vi "Pagina diagnostica.vi"(3 "error in (no error)":errorcluster) -> (9 "pagina out":i16=255, 10 "error out (no error)":errorcluster)   [LabVIEW 2022 SP3]
uses:
  <vilib>/Platform/TimedLoop/XDataNode/timing_clust.ctl
  <vilib>/Platform/TimedLoop/XDataNode/nitl_modes.ctl
  <vilib>/Platform/TimedLoop/XDataNode/wakeup.ctl
  Labview/Globali.vi
  <vilib>/platform/TimedLoop/XDataNode/XDataNode.xnode
  <vilib>/Platform/TimedLoop/XDataNode/XDNodeRunTimeDep.lvlib
panel:
  in  "226. 0":sgl min=0 format="%.2f"
  in  "230. 0":sgl min=0 format="%.2f"
  in  "Verniciato":bool
  out "CICLO_IN_CORSO":bool
  out "S_SCARTO":bool
  out "S_PAUSA":bool
  out "Cicli_macchina":u16
  in  "2. 8":bool
  in  "2. 7":bool
  out "S_CANCELLI_APERTI":bool
  out "S_CANCELLI_CHIUSI":bool
  out "S_CANCELLO_CHIUSURA":bool
  out "S_CANCELLO_APERTURA":bool
  out "V_SOVRAPRESSIONE_DX":sgl format="%.2f"
  out "V_SOVRAPRESSIONE_SX":sgl format="%.2f"
  out "CALIBRAZIONE_TORSIOMETRO":bool
  in  "2. 6":bool
  out "S_CARRO_IN_POSIZ_RP3000":bool
  out "S_FILTRO_INTASATO_PROT35":bool
  out "S_FILTRO_INTASATO_RICIRC":bool
  in  "2. 5":bool
  out "S_CANCELLO_DX_APERTO":bool
  out "S_CANCELLO_SX_CHIUSO":bool
  out "S_CANCELLO_DX_CHIUSO":bool
  out "S_AUX_ON":bool
  out "S_PRESSOSTATO_ARIA":bool
  out "S_CANCELLO_SX_APERTO":bool
  out "S_CANCELLO_SX_SBLOCCATO":bool
  out "S_CANCELLO_DX_SBLOCCATO":bool
  out "S_TRAZIONE_INSERITA":bool
  out "S_SCARICO_A_LAV":bool
  out "S_SCARICO_A_RIP":bool
  out "S_CARRELLO_10W30":bool
  out "S_CARRELLO_W90":bool
  out "S_CARRELLO_PROT35":bool
  out "S_SCARICO_B_LAV":bool
  out "S_SCARICO_B_RIP":bool
  out "S_CARRO_IN_POSIZ_AAT":bool
  out "S_MOTORE_FERMO":bool
  out "C_APERTURA_CANCELLI":bool
  out "C_START_PROVA":bool
  out "C_RESET":bool
  out "C_CHIUSURA_CANCELLI":bool
  out "C_FASE_SUCCESSIVA":bool
  out "S_ALLARME_INVERTER":bool
  out "S_LIVELLO_MIN_10W30":bool
  out "S_LIVELLO_MIN_W90":bool
  out "S_LIVELLO_MIN_PROT35":bool
  out "S_FILTRO_INTASATO_10W30":bool
  out "S_FILTRO_INTASATO_W90":bool
  out "S_PERDITA_10W30":bool
  out "S_PERDITA_W90":bool
  out "S_PERDITA_PROT35":bool
  out "S_TERMICA_10W30":bool
  out "S_TERMICA_W90":bool
  out "S_TERMICA_PROT35":bool
  out "S_TERMICA_RICIRCOLO":bool
  out "CARICO_ARIA_6_BAR":bool
  out "SCARICO_ARIA_6_BAR":bool
  out "CARICO_PRESSURIZZ":bool
  out "S_PERDITA_VASCA_RACCOLT":bool
  out "SCARICO_PRESSURIZZ":bool
  out "RICIRCOLO_OLIO":bool
  out "ACCENSIONE_AZIONAMENTO":bool
  out "START_MOTORE":bool
  out "POMPA_RICIRCOLO":bool
  out "SCARICO_B":bool
  out "EROGAZIONE_10W30":bool
  out "EROGAZIONE_W90":bool
  out "CHIUSURA_CANCELLI":bool
  out "APERTURA_CANCELLI":bool
  out "SCARICO_A":bool
  out "EROGAZIONE_PROT35":bool
  out "ROTAZIONE_SX":bool
  out "SBLOCCO_CANCELLI":bool
  out "LAMPADA_TRAZIONE_ON":bool
  out "POMPA_10W30":bool
  out "POMPA_W90":bool
  out "POMPA_PROT35":bool
  out "LAMPADA_ROSSA":bool
  out "LAMPADA_GIALLA":bool
  out "LAMPADA_VERDE":bool
  out "CICALINO":bool
  out "S_MAN":bool
  out "S_AUTO":bool
  out "mA_RICIRCOLO_OK":bool
  out "mA_RISCALDAMENTO_OK":bool
  out "mA_PRESS_INSERZ_ASSE_OK":bool
  out "mA_TRAZIONE_INSERITA":bool
  out "mA_TRAZIONE_DISINSERITA":bool
  out "mA_RODAGGIO_OK":bool
  out "mA_COPPIA_1_FUN_OK":bool
  out "mA_RICIRCOLO_1_FUN_OK":bool
  out "mA_COPPIA_2_FUN_OK":bool
  out "mA_RICIRCOLO_2_FUN_OK":bool
  out "mA_COPPIA_3_FUN_OK":bool
  out "S_ALLARME":bool
  out "mA_RICIRCOLO_3_FUN_OK":bool
  out "mA_GONFIAGGIO_OK":bool
  out "mA_PERDITE_DX_OK":bool
  out "mA_PERDITE_SX_OK":bool
  out "mA_COPPIA_4_FUN_OK":bool
  out "mA_RICIRCOLO_4_FUN_OK":bool
  out "mA_COPPIA_5_FUN_OK":bool
  out "mA_RICIRCOLO_5_FUN_OK":bool
  out "mA_PRESS_PRESSURIZZ_OK":bool
  out "mA_PRESSURIZZ_DX_OK":bool
  out "mA_PRESSURIZZ_SX_OK":bool
  out "Messaggi":u16
  out "Segnalazioni":u16
  out "Allarmi":u16
  out "Fase_collaudo":u16
  out "V_PORT_RICIRC_4_FUN_AAT2":sgl format="%.2f"
  out "V_PRES_OLIO_RICIRC_4_FUN":sgl format="%.2f"
  out "V_TEMP_CUSCIN_4_FUN_AAT":sgl format="%.2f"
  out "V_COPPIA_4_FUN":sgl format="%.2f"
  out "V_TEMP_OLIO_4_FUN":sgl format="%.2f"
  out "V_PORT_RICIRC_2_FUN_AAT2":sgl format="%.2f"
  out "V_PRES_OLIO_RICIRC_2_FUN":sgl format="%.2f"
  out "V_TEMP_CUSCIN_2_FUN_AAT":sgl format="%.2f"
  out "V_COPPIA_2_FUN":sgl format="%.2f"
  out "V_TEMP_OLIO_2_FUN":sgl format="%.2f"
  out "V_PERDITA_PRESSURIZZ_SX":sgl format="%.2f"
  out "V_PERDITA_PRESSURIZZ_DX":sgl format="%.2f"
  out "V_PERDITA_GONFIAGGIO_SX":sgl format="%.2f"
  out "V_PERDITA_GONFIAGGIO_DX":sgl format="%.2f"
  out "V_PRESS_PRESSURIZZ":sgl format="%.2f"
  out "V_PORT_RICIRC_5_FUN_AAT2":sgl format="%.2f"
  out "V_PRES_OLIO_RICIRC_5_FUN":sgl format="%.2f"
  out "V_TEMP_CUSCIN_5_FUN_AAT":sgl format="%.2f"
  out "V_COPPIA_5_FUN":sgl format="%.2f"
  out "V_TEMP_OLIO_5_FUN":sgl format="%.2f"
  out "V_PORT_RICIRC_3_FUN_AAT2":sgl format="%.2f"
  out "V_PRES_OLIO_RICIRC_3_FUN":sgl format="%.2f"
  out "V_TEMP_CUSCIN_3_FUN_AAT":sgl format="%.2f"
  out "V_COPPIA_3_FUN":sgl format="%.2f"
  out "V_TEMP_OLIO_3_FUN":sgl format="%.2f"
  out "V_PORT_RICIRC_1_FUN_AAT2":sgl format="%.2f"
  out "V_PRES_OLIO_RICIRC_1_FUN":sgl format="%.2f"
  out "V_TEMP_CUSCIN_1_FUN_AAT":sgl format="%.2f"
  out "V_COPPIA_1_FUN":sgl format="%.2f"
  out "V_TEMP_OLIO_1_FUN":sgl format="%.2f"
  out "V_TEMP_OLIO_10W90":sgl format="%.2f"
  out "V_TEMP_OLIO_10W30":sgl format="%.2f"
  out "V_TEMP_OLIO_RP3000":sgl format="%.2f"
  out "V_TEMP_OLIO_AAT_1_3_4":sgl format="%.2f"
  out "V_TEMP_OLIO_AAT_2":sgl format="%.2f"
  out "V_TEMP_OLIO_ROD":sgl format="%.2f"
  out "V_GONFIAGGIO_STAB":sgl format="%.2f"
  out "VI_COPPIA_MOT":u16
  out "VO_VEL_MOT":u16
  out "VI_VEL_MOT":u16
  out "V_COPPIA_ASSE_TRASCINAM":sgl format="%.2f"
  out "V_PORTATA_RICIRCOLO":sgl format="%.2f"
  out "V_PRESS_OLIO_RICIRCOLO":sgl format="%.2f"
  out "V_PRESSURIZZAZIONE":sgl format="%.2f"
  out "V_PRESS_ARIA_6_BAR":sgl format="%.2f"
  out "V_TEMP_CUSCINETTO_AAT":sgl format="%.2f"
  out "V_TEMP_AMBIENTE":sgl format="%.2f"
  in  "0. 0":bool
  in  "0. 1":bool
  in  "0. 2":bool
  in  "0. 3":bool
  in  "0. 4":bool
  in  "0. 5":bool
  in  "0. 6":bool
  in  "0. 7":bool
  in  "1. 0":bool
  in  "1. 1":bool
  in  "1. 2":bool
  in  "1. 3":bool
  in  "1. 4":bool
  in  "1. 5":bool
  in  "1. 6":bool
  in  "1. 7":bool
  in  "2. 0":bool
  in  "2. 1":bool
  in  "2. 2":bool
  in  "2. 3":bool
  in  "2. 4":bool
  in  "4. 0":i16(ring) items=["PRODOTTO", "RP3000", "AAT 2", "AAT 1 3 4"]
  in  "6. 0":i16(ring) items=["TIPO", "PRODUZIONE", "RICAMBIO"]
  in  "8. 0":i16 min=0 max=3000
  in  "12. 0":sgl min=0 format="%.2f"
  in  "16. 0":i16 min=0
  in  "22. 0":sgl min=0 format="%.2f"
  in  "26. 0":sgl min=0 format="%.2f"
  in  "32. 0":sgl min=0 format="%.2f"
  in  "36. 0":sgl min=0 format="%.2f"
  in  "44. 0":i16 min=0
  in  "50. 0":i16 min=0
  in  "56. 0":i16 min=0
  in  "62. 0":i16 min=0
  in  "68. 0":i16 min=0
  in  "72. 0":sgl min=0 format="%.2f"
  in  "76. 0":sgl min=0 format="%.2f"
  in  "80. 0":sgl min=0 format="%.2f"
  in  "84. 0":i16 min=0
  in  "88. 0":sgl min=0 format="%.2f"
  in  "92. 0":sgl min=0 format="%.2f"
  in  "96. 0":sgl min=0 format="%.2f"
  in  "100. 0":i16 min=0
  in  "104. 0":sgl min=0 format="%.2f"
  in  "108. 0":sgl min=0 format="%.2f"
  in  "112. 0":sgl min=0 format="%.2f"
  in  "116. 0":i16 min=0
  in  "120. 0":sgl min=0 format="%.2f"
  in  "124. 0":sgl min=0 format="%.2f"
  in  "128. 0":sgl min=0 format="%.2f"
  in  "134. 0":sgl min=0 format="%.2f"
  in  "138. 0":sgl min=0 format="%.2f"
  in  "144. 0":i16 min=0
  in  "148. 0":i16 min=0
  in  "154. 0":i16 min=0
  in  "160. 0":sgl min=0 format="%.2f"
  in  "164. 0":sgl min=0 format="%.2f"
  in  "168. 0":sgl min=0 format="%.2f"
  in  "172. 0":i16 min=0
  in  "176. 0":sgl min=0 format="%.2f"
  in  "180. 0":sgl min=0 format="%.2f"
  in  "184. 0":sgl min=0 format="%.2f"
  in  "190. 0":sgl min=0 format="%.2f"
  in  "194. 0":sgl min=0 format="%.2f"
  in  "200. 0":i16 min=0
  in  "206. 0":i16 min=0
  in  "212. 0":i16 min=0
  in  "20. 0":u16
  in  "30. 0":u16
  in  "40. 0":u16
  in  "42. 0":u16
  in  "48. 0":u16
  in  "54. 0":u16
  in  "60. 0":u16
  in  "66. 0":u16
  in  "132. 0":u16
  in  "142. 0":u16
  in  "152. 0":u16
  in  "158. 0":u16
  in  "188. 0":u16
  in  "198. 0":u16
  in  "204. 0":u16
  in  "210. 0":u16
  in  "216. 0":u16
  in  "218. 0":u16
  out "PLC->PC":string[][](table)=[["WORD 0", "", "WORD 32", "", "WORD 64", "", "WORD 96", ""], ["WORD 1", "", "WORD 33", "", "WORD 65", "", "WORD 97", ""], ["WORD 2", "", "WORD 34", "", "WORD 66", "", "WORD 98", ""], ["WORD 3", "", "WORD 35", "", "WORD 67", "", "WORD 99", ""], ["WORD 4", "", "WORD 36", "", "WORD 68", "", "WORD 100", ""], ["WORD 5", "", "WORD 37", "", "WORD 69", "", "WORD 101", ""], ["WORD 6", "", "WORD 38", "", "WORD 70", "", "WORD 102", ""], ["WORD 7", "", "WORD 39", "", "WORD 71", "", "WORD 103", ""], ["WORD 8", "", "WORD 40", "", "WORD 72", "", "WORD 104", ""], ["WORD 9", "", "WORD 41", "", "WORD 73", "", "WORD 105", ""], ["WORD 10", "", "WORD 42", "", "WORD 74", "", "WORD 106", ""], ["WORD 11", "", "WORD 43", "", "WORD 75", "", "WORD 107", ""], ["WORD 12", "", "WORD 44", "", "WORD 76", "", "WORD 108", ""], ["WORD 13", "", "WORD 45", "", "WORD 77", "", "WORD 109", ""], ["WORD 14", "", "WORD 46", "", "WORD 78", "", "WORD 110", ""], ["WORD 15", "", "WORD 47", "", "WORD 79", "", "WORD 111", ""], ["WORD 16", "", "WORD 48", "", "WORD 80", "", "WORD 112", ""], ["WORD 17", "", "WORD 49", "", "WORD 81", "", "WORD 113", ""], ["WORD 18", "", "WORD 50", "", "WORD 82", "", "WORD 114", ""], ["WORD 19", "", "WORD 51", "", "WORD 83", "", "WORD 115", ""], ["WORD 20", "", "WORD 52", "", "WORD 84", "", "WORD 116", ""], ["WORD 21", "", "WORD 53", "", "WORD 85", "", "WORD 117", ""], ["WORD 22", "", "WORD 54", "", "WORD 86", "", "WORD 118", ""], ["WORD 23", "", "WORD 55", "", "WORD 87", "", "WORD 119", ""], ["WORD 24", "", "WORD 56", "", "WORD 88", "", "WORD 120", ""], ["WORD 25", "", "WORD 57", "", "WORD 89", "", "WORD 121", ""], ["WORD 26", "", "WORD 58", "", "WORD 90", "", "WORD 122", ""], ["WORD 27", "", "WORD 59", "", "WORD 91", "", "WORD 123", ""], ["WORD 28", "", "WORD 60", "", "WORD 92", "", "WORD 124", ""], ["WORD 29", "", "WORD 61", "", "WORD 93", "", "WORD 125", ""], ["WORD 30", "", "WORD 62", "", "WORD 94", "", "WORD 126", ""], ["WORD 31", "", "WORD 63", "", "WORD 95", "", "WORD 127", ""], ["", "", "", "", "", "", "", ""], ["", "", "", "", "", "", "", ""], ["", "", "", "", "", "", "", ""], ["", "", "", "", "", "", "", ""], ["", "", "", "", "", "", "", ""], ["", "", "", "", "", "", "", ""], ["", "", "", "", "", "", "", ""], ["", "", "", "", "", "", "", ""], ["", "", "", "", "", "", "", ""], ["", "", "", "", "", "", "", ""], ["", "", "", "", "", "", "", ""], ["", "", "", "", "", "", "", ""], ["", "", "", "", "", "", "", ""], ["", "", "", "", "", "", "", ""], ["", "", "", "", "", "", "", ""], ["", "", "", "", "", "", "", ""], ["", "", "", "", "", "", "", ""], ["", "", "", "", "", "", "", ""], ["", "", "", "", "", "", "", ""], ["", "", "", "", "", "", "", ""], ["", "", "", "", "", "", "", ""], ["", "", "", "", "", "", "", ""], ["", "", "", "", "", "", "", ""], ["", "", "", "", "", "", "", ""], ["", "", "", "", "", "", "", ""], ["", "", "", "", "", "", "", ""], ["", "", "", "", "", "", "", ""], ["", "", "", "", "", "", "", ""], ["", "", "", "", "", "", "", ""], ["", "", "", "", "", "", "", ""], ["", "", "", "", "", "", "", ""], ["", "", "", "", "", "", "", ""], ["", "", "", "", "", "", "", ""], ["", "", "", "", "", "", "", ""], ["", "", "", "", "", "", "", ""], ["", "", "", "", "", "", "", ""], ["", "", "", "", "", "", "", ""], ["", "", "", "", "", "", "", ""], ["", "", "", "", "", "", "", ""], ["", "", "", "", "", "", "", ""], ["", "", "", "", "", "", "", ""], ["", "", "", "", "", "", "", ""], ["", "", "", "", "", "", "", ""], ["", "", "", "", "", "", "", ""], ["", "", "", "", "", "", "", ""], ["", "", "", "", "", "", "", ""], ["", "", "", "", "", "", "", ""], ["", "", "", "", "", "", "", ""], ["", "", "", "", "", "", "", ""], ["", "", "", "", "", "", "", ""], ["", "", "", "", "", "", "", ""], ["", "", "", "", "", "", "", ""], ["", "", "", "", "", "", "", ""], ["", "", "", "", "", "", "", ""], ["", "", "", "", "", "", "", ""], ["", "", "", "", "", "", "", ""], ["", "", "", "", "", "", "", ""], ["", "", "", "", "", "", "", ""], ["", "", "", "", "", "", "", ""], ["", "", "", "", "", "", "", ""], ["", "", "", "", "", "", "", ""], ["", "", "", "", "", "", "", ""], ["", "", "", "", "", "", "", ""], ["", "", "", "", "", "", "", ""], ["", "", "", "", "", "", "", ""], ["", "", "", "", "", "", "", ""], ["", "", "", "", "", "", "", ""], ["", "", "", "", "", "", "", ""], ["", "", "", "", "", "", "", ""], ["", "", "", "", "", "", "", ""], ["", "", "", "", "", "", "", ""], ["", "", "", "", "", "", "", ""], ["", "", "", "", "", "", "", ""], ["", "", "", "", "", "", "", ""], ["", "", "", "", "", "", "", ""], ["", "", "", "", "", "", "", ""], ["", "", "", "", "", "", "", ""], ["", "", "", "", "", "", "", ""], ["", "", "", "", "", "", "", ""], ["", "", "", "", "", "", "", ""], ["", "", "", "", "", "", "", ""], ["", "", "", "", "", "", "", ""], ["", "", "", "", "", "", "", ""], ["", "", "", "", "", "", "", ""], ["", "", "", "", "", "", "", ""], ["", "", "", "", "", "", "", ""], ["", "", "", "", "", "", "", ""], ["", "", "", "", "", "", "", ""], ["", "", "", "", "", "", "", ""], ["", "", "", "", "", "", "", ""], ["", "", "", "", "", "", "", ""], ["", "", "", "", "", "", "", ""], ["", "", "", "", "", "", "", ""], ["", "", "", "", "", "", "", ""], ["", "", "", "", "", "", "", ""], ["", "", "", "", "", "", "", ""]]
  in  "Uscita":bool
  out "Errore conn. centralina":string="PAGINA DIAGNOSTICA" caption="Collaudo in corso"
  out "Collaudo in corso":string
  in  "stop":bool
  out "Versione SW":dbl=1.0 format="%.2f"
  # "PC->PLC"
  # "K_VEL_MOT_MAN"
  # "KT_3_ROD"
  # "K_TEMP_OLIO_3_FUN"
  # "K_TEMP_OLIO_5_FUN"
  # "K_TEMP_OLIO_RP_RISC"
  # "K_VEL_MOT_4_ROD"
  # "K_COPPIA_3_FUN_MIN"
  # "K_COPPIA_5_FUN_MIN"
  # "K_VEL_MOT_RISC"
  # "KT_4_ROD"
  # "K_COPPIA_3_FUN_MAX"
  # "K_COPPIA_5_FUN_MAX"
  # "KT_RISCALDO_AAT"
  # "K_VEL_MOT_5_ROD"
  # "KT_GONFIAGGIO"
  # "KT_PRESSURIZZAZIONE"
  # "K_PRESS_OLIO_RICIRC_MIN"
  # "K_TEMP_OLIO_ROD"
  # "K_PRESS_GONFIAGGIO_MIN"
  # "K_PRESSURIZZAZIONE_MIN"
  # "K_PRESS_OLIO_RICIRC_MAX"
  # "K_PRESS_RICIRC_MIN"
  # "K_PRESS_GONFIAGGIO_MAX"
  # "K_PRESSURIZZAZIONE_MAX"
  # "KT_PRESSURIZZ_INSERZIONE"
  # "K_PRESS_RICIRC_MAX"
  # "KT_STABILIZZ_GONFIAGGIO"
  # "KT_STABILIZZ_PRESSURIZZ"
  # "K_PRESS_INSERZ_ASSE_MIN"
  # "K_VEL_MOT_1_FUN"
  # "K_VEL_MOT_4_FUN_RP_DX"
  # "K_VEL_PRESSURIZZ_DX"
  # "K_PRESS_INSERZ_ASSE_MAX"
  # "K_TEMP_OLIO_1_FUN"
  # "K_VEL_MOT_4_FUN"
  # "KT_PRESSURIZZ_DX"
  # "KT_INSERZIONE_1_ASSE"
  # "K_COPPIA_1_FUN_MIN"
  # "KT_4_FUN_RP_DX"
  # "K_VEL_PRESSURIZZ_SX"
  # "KT_DISINSERZIONE_1_ASSE"
  # "K_COPPIA_1_FUN_MAX"
  # "K_VEL_MOT_4_FUN_RP_SX"
  # "KT_PRESSURIZZ_SX"
  # "K_VEL_MOT_1_ROD"
  # "K_VEL_MOT_2_FUN"
  # "KT_4_FUN_RP_SX"
  # "K_VEL_MOT_PROT35"
  # "KT_1_ROD"
  # "K_TEMP_OLIO_2_FUN"
  # "K_TEMP_OLIO_4_FUN"
  # "KT_PROT35_SX"
  # "K_VEL_MOT_2_ROD"
  # "K_COPPIA_2_FUN_MIN"
  # "K_COPPIA_4_FUN_MIN"
  # "KT_PROT35_DX"
  # "KT_2_ROD"
  # "K_COPPIA_2_FUN_MAX"
  # "K_COPPIA_4_FUN_MAX"
  # "K_PERD_GONFIAGGIO"
  # "K_VEL_MOT_3_ROD"
  # "K_VEL_MOT_3_FUN"
  # "K_VEL_MOT_5_FUN"
  # "K_PERD_PRESSURIZZ"
  # "PLC->PC"
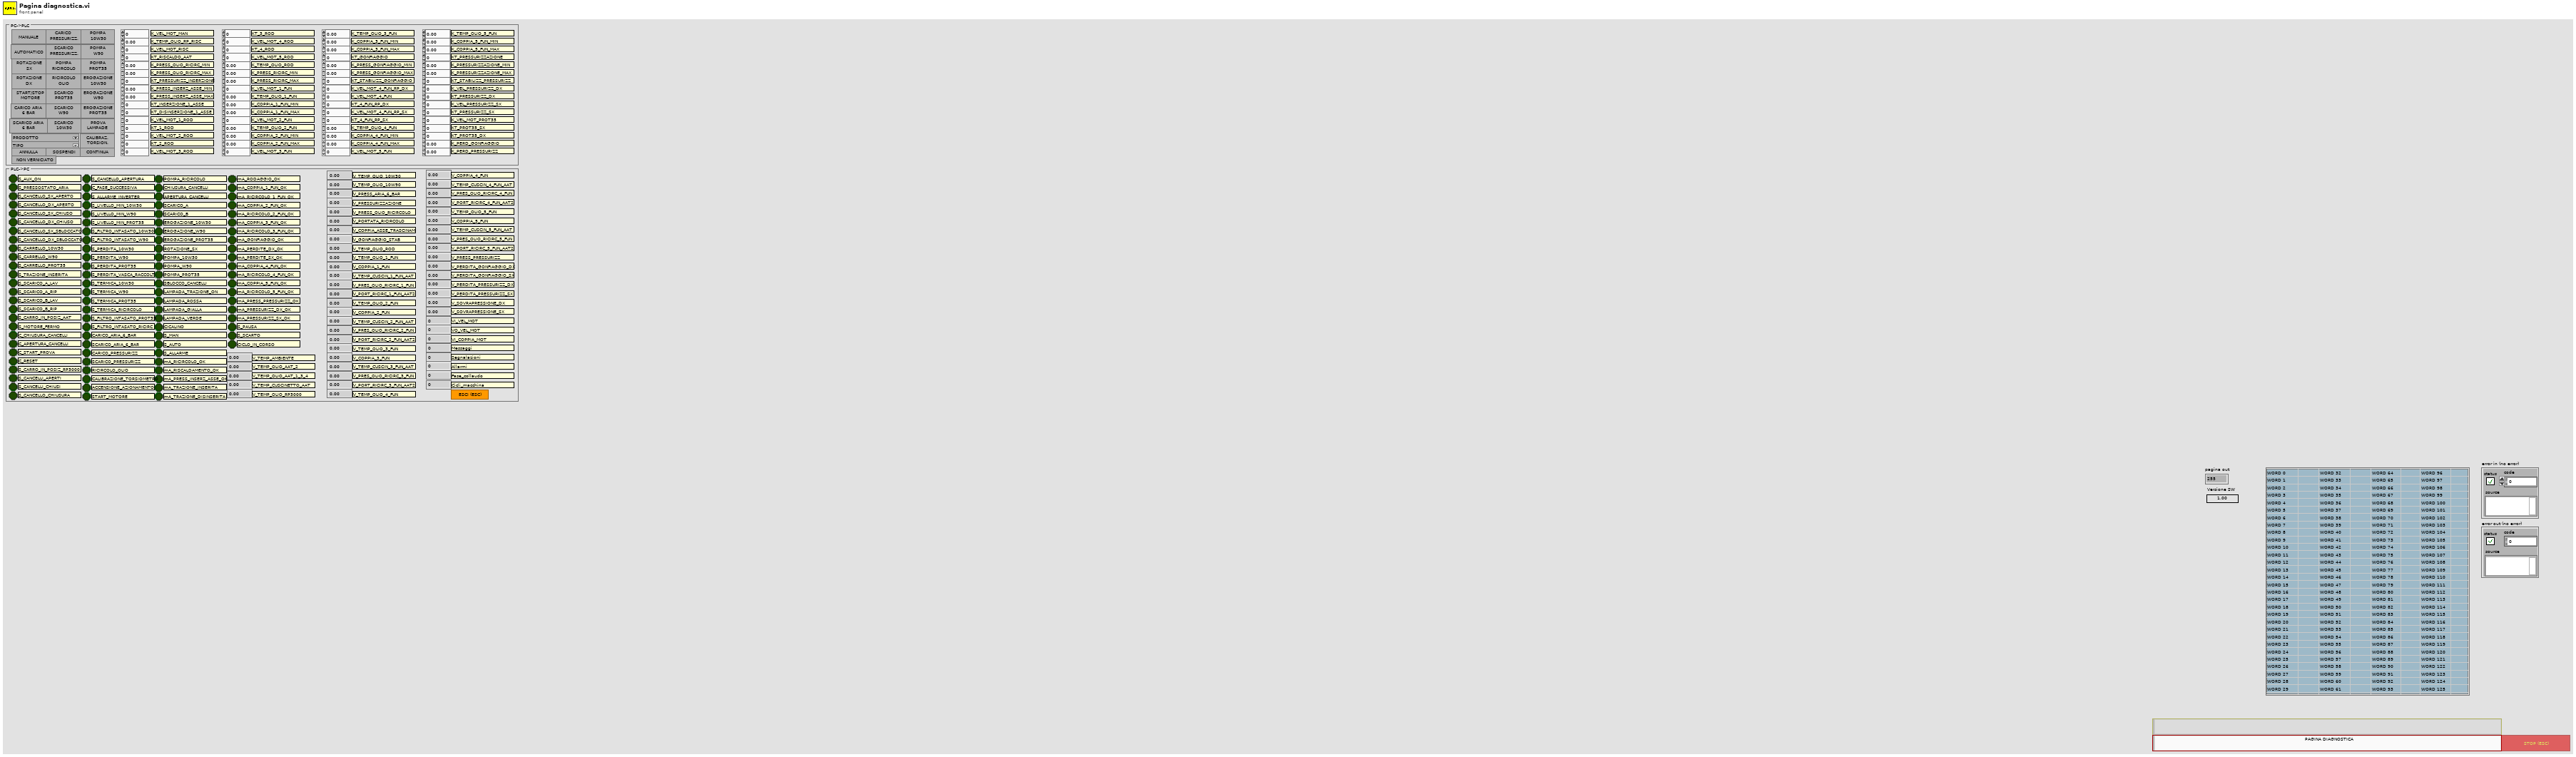
[diagram p1: front panel]
types:
  T1 = typedef "XDNodeRunTimeDep.lvlib/timing_clust.ctl" = cluster{"Expected End [f-1]":u64, "Actual End [f-1]":u64, "Finished Late? [f-1]":bool, "Expected End [i-1]":u64, "Actual End [i-1]":u64, "Finished Late? [i-1]":bool, "Expected Start [i]":u64, "Actual Start [i]":u64, "Expected Start [f]":u64, "Actual Start [f]":u64, "Source Name":string, "Structure Name":string, "Period":i64, "Deadline":i64, "Offset":i64, "Start":i64, "Priority":i32, "Timeout":i32, "Mode":T2, "Wakeup Reason":T3, "Error":errorcluster, "Source Type":string, "Secondary Source Type":string, "Global End Time":u64, "Global Start Time":u64, "Frame Duration":u64, "Iteration Duration":u64, "Assigned CPU":i32, "I/O Scan Engine Mode":u32}
  T2 = typedef "XDNodeRunTimeDep.lvlib/nitl_modes.ctl" = enum32{"No Change", "Process missed periods, maintain original phase", "Discard missed periods, maintain original phase", "Process missed periods, ignore original phase", "Discard missed periods, ignore original phase"}
  T3 = typedef "XDNodeRunTimeDep.lvlib/wakeup.ctl" = enum32{"Normal", "Aborted", "Asynchronous wakeup", "Timing source error", "Timed loop error", "Timeout"}
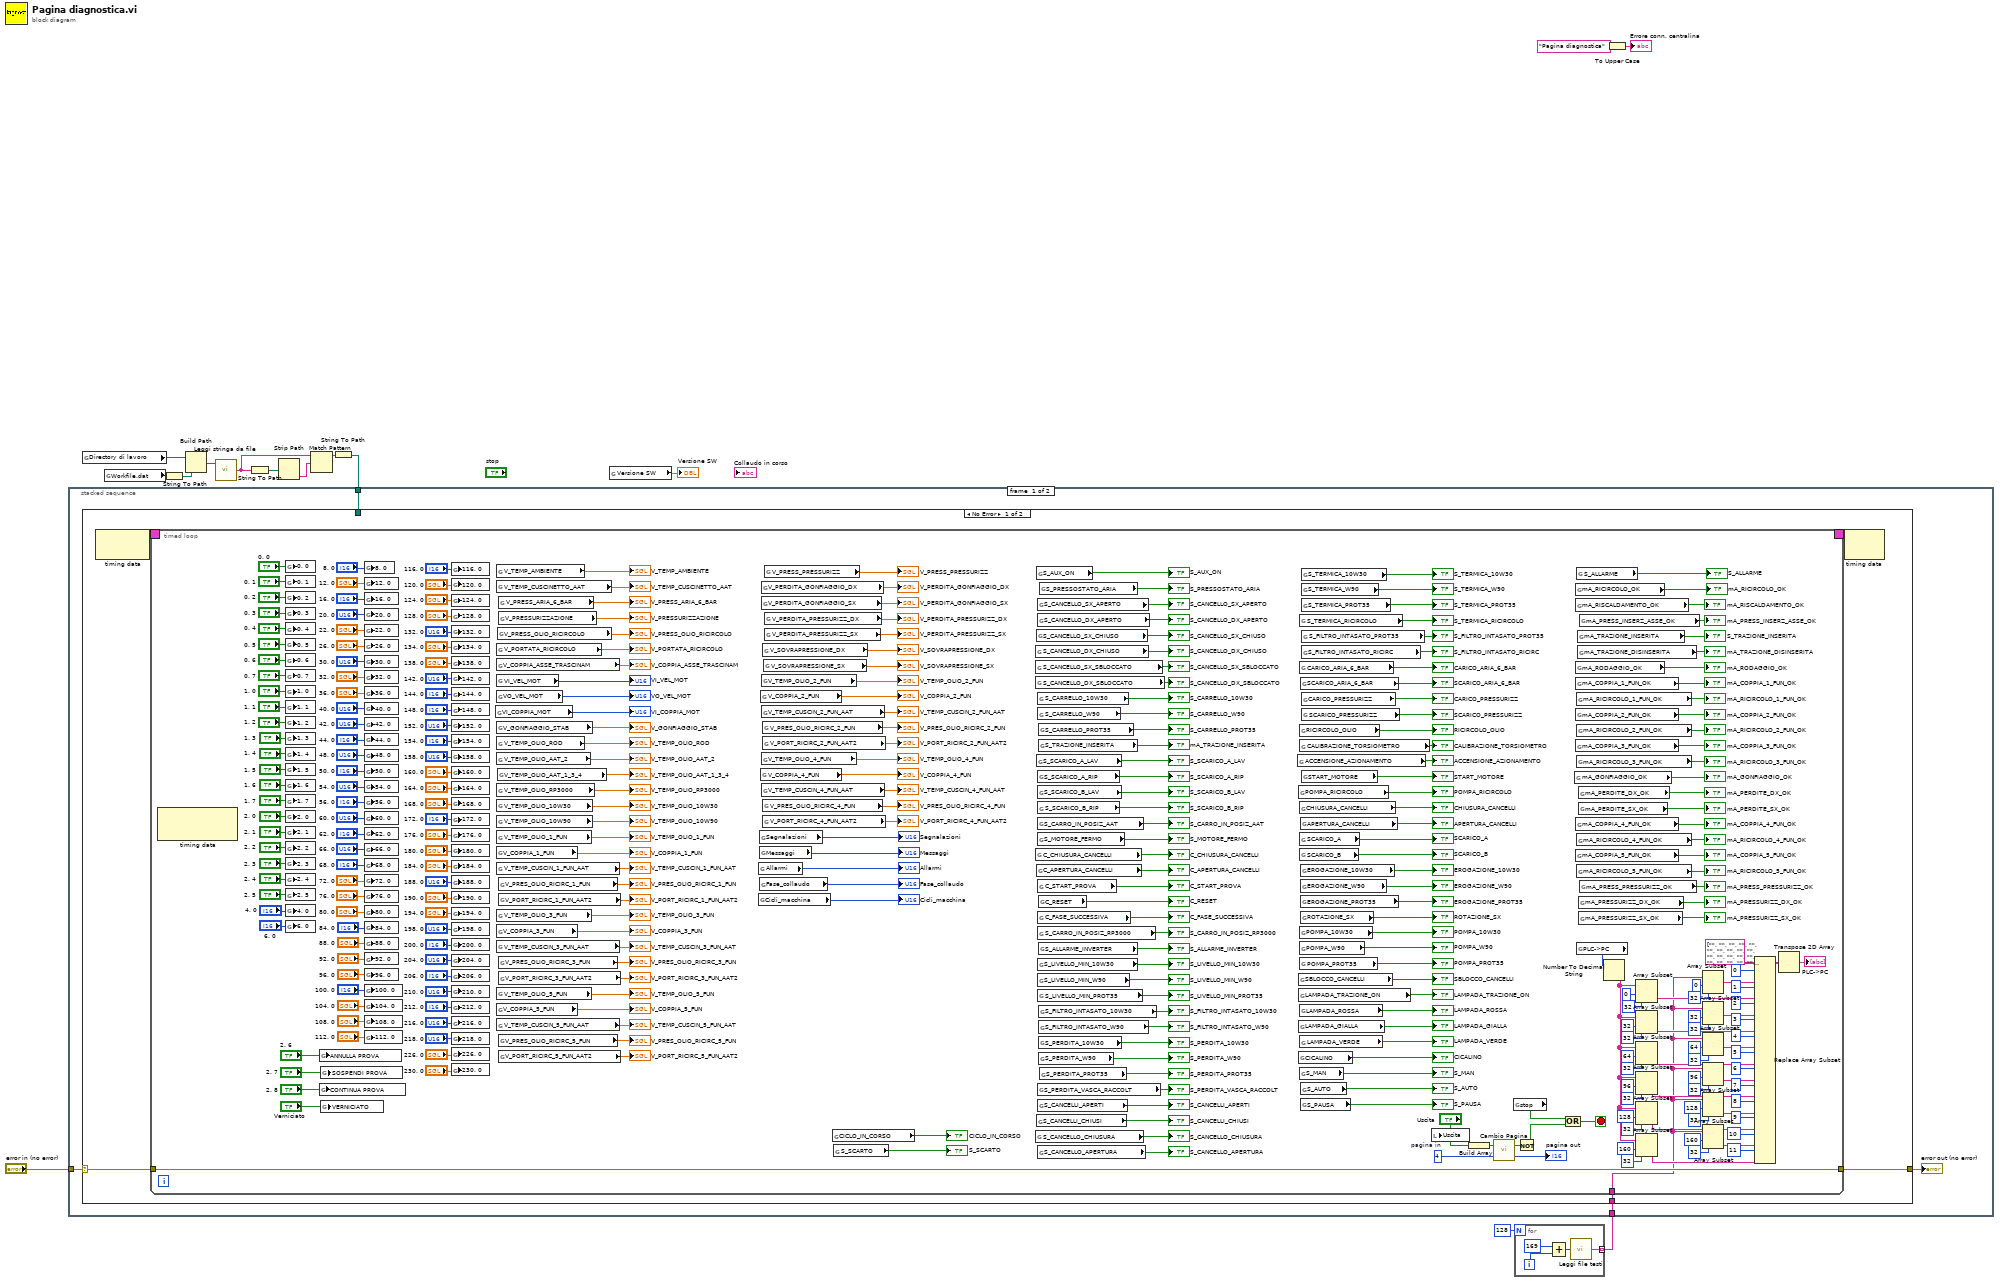
[diagram p0: block diagram]
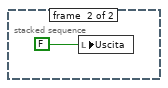
[diagram p3: hidden frame]
diagram:
  n1 = global read "Globali.vi" "Directory di lavoro"() -> (w10:path)
  n2 = global read "Globali.vi" "Workfile.dat"() -> (w9:string)
  n3 = String To Path(string=w9) -> (path=w12:path)
  n4 = Build Path(base path=w10, name or relative path=w12) -> (appended path=w11:path)
  n5 = call "Leggi stringa da file.vi"("file path (dialog if empty)"=w11) -> ("character string"=w5:string)  [unwired: 5 in, 3 out]
  n6 = String To Path(string=w5) -> (path=w8:path)
  n7 = Strip Path(path=w8) -> (name=w7:string)  [unwired: 1 out]
  n8 = Match Pattern(string=w5, regular expression=w7) -> (before substring=w6:string)  [unwired: 1 in, 3 out]
  n9 = String To Path(string=w6) -> (path=w4:path)
  n10 = global read "globali.vi" "Versione SW"() -> (→"Versione SW":dbl)
  n11 = for {
    N: 128 -> [_]
    tunnel: [w17] -> w1 mode=indexing
    i -> [w16]
    n12 = Add(x=169, y=w16) -> (x+y=w19:i32)
    n13 = call "Leggi file testi.vi"("Numero riga"=w19) -> ("Testo"=w17:string)  [unwired: 3 in, 1 out]
  }
  n14 = stacked-sequence {
    tunnel: "error in (no error)" -> [w23 _]
    tunnel: w4 -> [w21 _]
    tunnel: w1 -> [w20 _]
    frame #0 {
      n15 = case shown="No Error" w23 {
        selector: w23 -> [w27 w340]
        tunnel: [w28 w340] -> w22
        tunnel: w21 -> [_ _]
        tunnel: w20 -> [w26 _]
        frame No Error {
          n16 = node-c288() -> (w25:T1)  [unwired: 1 in]
          n17 = timed-loop {
            tunnel: w26 -> [w275]
            timing-out: [_] -> w24
            timing: w25 -> [_]
            tunnel: w27 -> [w333]
            tunnel: [w333] -> w28
            stop <- w334 stop-if-true
            w330 = u8 4  # pagina in
            n18 = node-c288() -> ()  [unwired: 1 in, 2 out]
            n19 = global write "Globali.vi" "0. 0"("0. 0") -> ()
            n20 = global write "Globali.vi" "0. 1"("0. 1") -> ()
            n21 = global write "Globali.vi" "0. 2"("0. 2") -> ()
            n22 = global write "Globali.vi" "0. 3"("0. 3") -> ()
            n23 = global write "Globali.vi" "0. 4"("0. 4") -> ()
            n24 = global write "Globali.vi" "0. 5"("0. 5") -> ()
            n25 = global write "Globali.vi" "0. 6"("0. 6") -> ()
            n26 = global write "Globali.vi" "0. 7"("0. 7") -> ()
            n27 = global write "Globali.vi" "1. 0"("1. 0") -> ()
            n28 = global write "Globali.vi" "1. 1"("1. 1") -> ()
            n29 = global write "Globali.vi" "1. 2"("1. 2") -> ()
            n30 = global write "Globali.vi" "1. 3"("1. 3") -> ()
            n31 = global write "Globali.vi" "1. 4"("1. 4") -> ()
            n32 = global write "Globali.vi" "1. 5"("1. 5") -> ()
            n33 = global write "Globali.vi" "1. 6"("1. 6") -> ()
            n34 = global write "Globali.vi" "1. 7"("1. 7") -> ()
            n35 = global write "Globali.vi" "2. 0"("2. 0") -> ()
            n36 = global write "Globali.vi" "2. 1"("2. 1") -> ()
            n37 = global write "Globali.vi" "2. 2"("2. 2") -> ()
            n38 = global write "Globali.vi" "2. 3"("2. 3") -> ()
            n39 = global write "Globali.vi" "2. 4"("2. 4") -> ()
            n40 = global write "Globali.vi" "2. 5"("2. 5") -> ()
            n41 = global write "Globali.vi" "4. 0"("4. 0") -> ()
            n42 = global write "Globali.vi" "6. 0"("6. 0") -> ()
            n43 = global write "Globali.vi" "ANNULLA PROVA"("2. 6") -> ()
            n44 = global write "Globali.vi" "CONTINUA PROVA"("2. 8") -> ()
            n45 = global write "Globali.vi" "SOSPENDI PROVA"("2. 7") -> ()
            n46 = global write "Globali.vi" "VERNICIATO"("Verniciato") -> ()
            n47 = global write "Globali.vi" "8. 0"("8. 0") -> ()
            n48 = global write "Globali.vi" "12. 0"("12. 0") -> ()
            n49 = global write "Globali.vi" "16. 0"("16. 0") -> ()
            n50 = global write "Globali.vi" "20. 0"("20. 0") -> ()
            n51 = global write "Globali.vi" "22. 0"("22. 0") -> ()
            n52 = global write "Globali.vi" "26. 0"("26. 0") -> ()
            n53 = global write "Globali.vi" "30. 0"("30. 0") -> ()
            n54 = global write "Globali.vi" "32. 0"("32. 0") -> ()
            n55 = global write "Globali.vi" "36. 0"("36. 0") -> ()
            n56 = global write "Globali.vi" "40. 0"("40. 0") -> ()
            n57 = global write "Globali.vi" "42. 0"("42. 0") -> ()
            n58 = global write "Globali.vi" "44. 0"("44. 0") -> ()
            n59 = global write "Globali.vi" "48. 0"("48. 0") -> ()
            n60 = global write "Globali.vi" "50. 0"("50. 0") -> ()
            n61 = global write "Globali.vi" "54. 0"("54. 0") -> ()
            n62 = global write "Globali.vi" "56. 0"("56. 0") -> ()
            n63 = global write "Globali.vi" "60. 0"("60. 0") -> ()
            n64 = global write "Globali.vi" "62. 0"("62. 0") -> ()
            n65 = global write "Globali.vi" "66. 0"("66. 0") -> ()
            n66 = global write "Globali.vi" "68. 0"("68. 0") -> ()
            n67 = global write "Globali.vi" "72. 0"("72. 0") -> ()
            n68 = global write "Globali.vi" "76. 0"("76. 0") -> ()
            n69 = global write "Globali.vi" "80. 0"("80. 0") -> ()
            n70 = global write "Globali.vi" "84. 0"("84. 0") -> ()
            n71 = global write "Globali.vi" "88. 0"("88. 0") -> ()
            n72 = global write "Globali.vi" "92. 0"("92. 0") -> ()
            n73 = global write "Globali.vi" "96. 0"("96. 0") -> ()
            n74 = global write "Globali.vi" "100. 0"("100. 0") -> ()
            n75 = global write "Globali.vi" "104. 0"("104. 0") -> ()
            n76 = global write "Globali.vi" "108. 0"("108. 0") -> ()
            n77 = global write "Globali.vi" "112. 0"("112. 0") -> ()
            n78 = global write "Globali.vi" "116. 0"("116. 0") -> ()
            n79 = global write "Globali.vi" "120. 0"("120. 0") -> ()
            n80 = global write "Globali.vi" "124. 0"("124. 0") -> ()
            n81 = global write "Globali.vi" "128. 0"("128. 0") -> ()
            n82 = global write "Globali.vi" "132. 0"("132. 0") -> ()
            n83 = global write "Globali.vi" "134. 0"("134. 0") -> ()
            n84 = global write "Globali.vi" "138. 0"("138. 0") -> ()
            n85 = global write "Globali.vi" "142. 0"("142. 0") -> ()
            n86 = global write "Globali.vi" "144. 0"("144. 0") -> ()
            n87 = global write "Globali.vi" "148. 0"("148. 0") -> ()
            n88 = global write "Globali.vi" "152. 0"("152. 0") -> ()
            n89 = global write "Globali.vi" "154. 0"("154. 0") -> ()
            n90 = global write "Globali.vi" "158. 0"("158. 0") -> ()
            n91 = global write "Globali.vi" "160. 0"("160. 0") -> ()
            n92 = global write "Globali.vi" "164. 0"("164. 0") -> ()
            n93 = global write "Globali.vi" "168. 0"("168. 0") -> ()
            n94 = global write "Globali.vi" "172. 0"("172. 0") -> ()
            n95 = global write "Globali.vi" "176. 0"("176. 0") -> ()
            n96 = global write "Globali.vi" "180. 0"("180. 0") -> ()
            n97 = global write "Globali.vi" "184. 0"("184. 0") -> ()
            n98 = global write "Globali.vi" "188. 0"("188. 0") -> ()
            n99 = global write "Globali.vi" "190. 0"("190. 0") -> ()
            n100 = global write "Globali.vi" "194. 0"("194. 0") -> ()
            n101 = global write "Globali.vi" "198. 0"("198. 0") -> ()
            n102 = global write "Globali.vi" "200. 0"("200. 0") -> ()
            n103 = global write "Globali.vi" "204. 0"("204. 0") -> ()
            n104 = global write "Globali.vi" "206. 0"("206. 0") -> ()
            n105 = global write "Globali.vi" "210. 0"("210. 0") -> ()
            n106 = global write "Globali.vi" "212. 0"("212. 0") -> ()
            n107 = global write "Globali.vi" "216. 0"("216. 0") -> ()
            n108 = global write "Globali.vi" "218. 0"("218. 0") -> ()
            n109 = global write "Globali.vi" "226. 0"("226. 0") -> ()
            n110 = global write "Globali.vi" "230. 0"("230. 0") -> ()
            n111 = global read "Globali.vi" "VI_COPPIA_MOT"() -> (→"VI_COPPIA_MOT":u16)
            n112 = global read "Globali.vi" "V_COPPIA_ASSE_TRASCINAM"() -> (→"V_COPPIA_ASSE_TRASCINAM":sgl)
            n113 = global read "Globali.vi" "VO_VEL_MOT"() -> (→"VO_VEL_MOT":u16)
            n114 = global read "Globali.vi" "V_GONFIAGGIO_STAB"() -> (→"V_GONFIAGGIO_STAB":sgl)
            n115 = global read "Globali.vi" "V_COPPIA_1_FUN"() -> (→"V_COPPIA_1_FUN":sgl)
            n116 = global read "Globali.vi" "V_COPPIA_3_FUN"() -> (→"V_COPPIA_3_FUN":sgl)
            n117 = global read "Globali.vi" "V_COPPIA_5_FUN"() -> (→"V_COPPIA_5_FUN":sgl)
            n118 = global read "Globali.vi" "V_TEMP_AMBIENTE"() -> (→"V_TEMP_AMBIENTE":sgl)
            n119 = global read "Globali.vi" "V_TEMP_CUSCINETTO_AAT"() -> (→"V_TEMP_CUSCINETTO_AAT":sgl)
            n120 = global read "Globali.vi" "V_PORTATA_RICIRCOLO"() -> (→"V_PORTATA_RICIRCOLO":sgl)
            n121 = global read "Globali.vi" "VI_VEL_MOT"() -> (→"VI_VEL_MOT":u16)
            n122 = global read "Globali.vi" "V_TEMP_OLIO_ROD"() -> (→"V_TEMP_OLIO_ROD":sgl)
            n123 = global read "Globali.vi" "V_TEMP_OLIO_AAT_2"() -> (→"V_TEMP_OLIO_AAT_2":sgl)
            n124 = global read "Globali.vi" "V_TEMP_OLIO_RP3000"() -> (→"V_TEMP_OLIO_RP3000":sgl)
            n125 = global read "Globali.vi" "V_TEMP_OLIO_10W30"() -> (→"V_TEMP_OLIO_10W30":sgl)
            n126 = global read "Globali.vi" "V_TEMP_OLIO_10W90"() -> (→"V_TEMP_OLIO_10W90":sgl)
            n127 = global read "Globali.vi" "V_TEMP_OLIO_1_FUN"() -> (→"V_TEMP_OLIO_1_FUN":sgl)
            n128 = global read "Globali.vi" "V_TEMP_CUSCIN_1_FUN_AAT"() -> (→"V_TEMP_CUSCIN_1_FUN_AAT":sgl)
            n129 = global read "Globali.vi" "V_TEMP_OLIO_3_FUN"() -> (→"V_TEMP_OLIO_3_FUN":sgl)
            n130 = global read "Globali.vi" "V_TEMP_CUSCIN_3_FUN_AAT"() -> (→"V_TEMP_CUSCIN_3_FUN_AAT":sgl)
            n131 = global read "Globali.vi" "V_TEMP_OLIO_5_FUN"() -> (→"V_TEMP_OLIO_5_FUN":sgl)
            n132 = global read "Globali.vi" "V_TEMP_CUSCIN_5_FUN_AAT"() -> (→"V_TEMP_CUSCIN_5_FUN_AAT":sgl)
            n133 = global read "Globali.vi" "V_PRESS_OLIO_RICIRCOLO"() -> (→"V_PRESS_OLIO_RICIRCOLO":sgl)
            n134 = global read "Globali.vi" "V_TEMP_OLIO_AAT_1_3_4"() -> (→"V_TEMP_OLIO_AAT_1_3_4":sgl)
            n135 = global read "Globali.vi" "V_PRESSURIZZAZIONE"() -> (→"V_PRESSURIZZAZIONE":sgl)
            n136 = global read "Globali.vi" "V_PRES_OLIO_RICIRC_1_FUN"() -> (→"V_PRES_OLIO_RICIRC_1_FUN":sgl)
            n137 = global read "Globali.vi" "V_PORT_RICIRC_1_FUN_AAT2"() -> (→"V_PORT_RICIRC_1_FUN_AAT2":sgl)
            n138 = global read "Globali.vi" "V_PRES_OLIO_RICIRC_3_FUN"() -> (→"V_PRES_OLIO_RICIRC_3_FUN":sgl)
            n139 = global read "Globali.vi" "V_PORT_RICIRC_3_FUN_AAT2"() -> (→"V_PORT_RICIRC_3_FUN_AAT2":sgl)
            n140 = global read "Globali.vi" "V_PRES_OLIO_RICIRC_5_FUN"() -> (→"V_PRES_OLIO_RICIRC_5_FUN":sgl)
            n141 = global read "Globali.vi" "V_PORT_RICIRC_5_FUN_AAT2"() -> (→"V_PORT_RICIRC_5_FUN_AAT2":sgl)
            n142 = global read "Globali.vi" "V_PRESS_ARIA_6_BAR"() -> (→"V_PRESS_ARIA_6_BAR":sgl)
            n143 = global read "Globali.vi" "Cicli_macchina"() -> (→"Cicli_macchina":u16)
            n144 = global read "Globali.vi" "Allarmi"() -> (→"Allarmi":u16)
            n145 = global read "Globali.vi" "Segnalazioni"() -> (→"Segnalazioni":u16)
            n146 = global read "Globali.vi" "Messaggi"() -> (→"Messaggi":u16)
            n147 = global read "Globali.vi" "Fase_collaudo"() -> (→"Fase_collaudo":u16)
            n148 = global read "Globali.vi" "V_COPPIA_2_FUN"() -> (→"V_COPPIA_2_FUN":sgl)
            n149 = global read "Globali.vi" "V_COPPIA_4_FUN"() -> (→"V_COPPIA_4_FUN":sgl)
            n150 = global read "Globali.vi" "V_PERDITA_GONFIAGGIO_DX"() -> (→"V_PERDITA_GONFIAGGIO_DX":sgl)
            n151 = global read "Globali.vi" "V_PERDITA_GONFIAGGIO_SX"() -> (→"V_PERDITA_GONFIAGGIO_SX":sgl)
            n152 = global read "Globali.vi" "V_TEMP_OLIO_2_FUN"() -> (→"V_TEMP_OLIO_2_FUN":sgl)
            n153 = global read "Globali.vi" "V_TEMP_CUSCIN_2_FUN_AAT"() -> (→"V_TEMP_CUSCIN_2_FUN_AAT":sgl)
            n154 = global read "Globali.vi" "V_TEMP_OLIO_4_FUN"() -> (→"V_TEMP_OLIO_4_FUN":sgl)
            n155 = global read "Globali.vi" "V_TEMP_CUSCIN_4_FUN_AAT"() -> (→"V_TEMP_CUSCIN_4_FUN_AAT":sgl)
            n156 = global read "Globali.vi" "V_SOVRAPRESSIONE_DX"() -> (→"V_SOVRAPRESSIONE_DX":sgl)
            n157 = global read "Globali.vi" "V_PRES_OLIO_RICIRC_2_FUN"() -> (→"V_PRES_OLIO_RICIRC_2_FUN":sgl)
            n158 = global read "Globali.vi" "V_PORT_RICIRC_2_FUN_AAT2"() -> (→"V_PORT_RICIRC_2_FUN_AAT2":sgl)
            n159 = global read "Globali.vi" "V_PRES_OLIO_RICIRC_4_FUN"() -> (→"V_PRES_OLIO_RICIRC_4_FUN":sgl)
            n160 = global read "Globali.vi" "V_PORT_RICIRC_4_FUN_AAT2"() -> (→"V_PORT_RICIRC_4_FUN_AAT2":sgl)
            n161 = global read "Globali.vi" "V_SOVRAPRESSIONE_SX"() -> (→"V_SOVRAPRESSIONE_SX":sgl)
            n162 = global read "Globali.vi" "V_PRESS_PRESSURIZZ"() -> (→"V_PRESS_PRESSURIZZ":sgl)
            n163 = global read "Globali.vi" "V_PERDITA_PRESSURIZZ_DX"() -> (→"V_PERDITA_PRESSURIZZ_DX":sgl)
            n164 = global read "Globali.vi" "V_PERDITA_PRESSURIZZ_SX"() -> (→"V_PERDITA_PRESSURIZZ_SX":sgl)
            n165 = global read "Globali.vi" "CICLO_IN_CORSO"() -> (→"CICLO_IN_CORSO":bool)
            n166 = global read "Globali.vi" "S_SCARTO"() -> (→"S_SCARTO":bool)
            n167 = global read "Globali.vi" "S_CANCELLO_DX_CHIUSO"() -> (→"S_CANCELLO_DX_CHIUSO":bool)
            n168 = global read "Globali.vi" "S_CANCELLO_SX_SBLOCCATO"() -> (→"S_CANCELLO_SX_SBLOCCATO":bool)
            n169 = global read "Globali.vi" "S_CANCELLO_DX_SBLOCCATO"() -> (→"S_CANCELLO_DX_SBLOCCATO":bool)
            n170 = global read "Globali.vi" "C_CHIUSURA_CANCELLI"() -> (→"C_CHIUSURA_CANCELLI":bool)
            n171 = global read "Globali.vi" "S_CANCELLO_CHIUSURA"() -> (→"S_CANCELLO_CHIUSURA":bool)
            n172 = global read "Globali.vi" "S_AUX_ON"() -> (→"S_AUX_ON":bool)
            n173 = global read "Globali.vi" "S_CANCELLO_SX_CHIUSO"() -> (→"S_CANCELLO_SX_CHIUSO":bool)
            n174 = global read "Globali.vi" "S_SCARICO_A_LAV"() -> (→"S_SCARICO_A_LAV":bool)
            n175 = global read "Globali.vi" "C_APERTURA_CANCELLI"() -> (→"C_APERTURA_CANCELLI":bool)
            n176 = global read "Globali.vi" "S_CANCELLI_CHIUSI"() -> (→"S_CANCELLI_CHIUSI":bool)
            n177 = global read "Globali.vi" "S_CANCELLO_SX_APERTO"() -> (→"S_CANCELLO_SX_APERTO":bool)
            n178 = global read "Globali.vi" "S_CANCELLO_DX_APERTO"() -> (→"S_CANCELLO_DX_APERTO":bool)
            n179 = global read "Globali.vi" "S_SCARICO_A_RIP"() -> (→"S_SCARICO_A_RIP":bool)
            n180 = global read "Globali.vi" "S_SCARICO_B_LAV"() -> (→"S_SCARICO_B_LAV":bool)
            n181 = global read "Globali.vi" "S_CARRO_IN_POSIZ_AAT"() -> (→"S_CARRO_IN_POSIZ_AAT":bool)
            n182 = global read "Globali.vi" "S_MOTORE_FERMO"() -> (→"S_MOTORE_FERMO":bool)
            n183 = global read "Globali.vi" "S_LIVELLO_MIN_10W30"() -> (→"S_LIVELLO_MIN_10W30":bool)
            n184 = global read "Globali.vi" "S_LIVELLO_MIN_W90"() -> (→"S_LIVELLO_MIN_W90":bool)
            n185 = global read "Globali.vi" "S_PERDITA_VASCA_RACCOLT"() -> (→"S_PERDITA_VASCA_RACCOLT":bool)
            n186 = global read "Globali.vi" "S_CANCELLI_APERTI"() -> (→"S_CANCELLI_APERTI":bool)
            n187 = global read "Globali.vi" "S_CANCELLO_APERTURA"() -> (→"S_CANCELLO_APERTURA":bool)
            n188 = global read "Globali.vi" "S_CARRELLO_10W30"() -> (→"S_CARRELLO_10W30":bool)
            n189 = global read "Globali.vi" "S_CARRELLO_W90"() -> (→"S_CARRELLO_W90":bool)
            n190 = global read "Globali.vi" "S_SCARICO_B_RIP"() -> (→"S_SCARICO_B_RIP":bool)
            n191 = global read "Globali.vi" "C_START_PROVA"() -> (→"C_START_PROVA":bool)
            n192 = global read "Globali.vi" "C_FASE_SUCCESSIVA"() -> (→"C_FASE_SUCCESSIVA":bool)
            n193 = global read "Globali.vi" "S_CARRO_IN_POSIZ_RP3000"() -> (→"S_CARRO_IN_POSIZ_RP3000":bool)
            n194 = global read "Globali.vi" "S_LIVELLO_MIN_PROT35"() -> (→"S_LIVELLO_MIN_PROT35":bool)
            n195 = global read "Globali.vi" "S_CARRELLO_PROT35"() -> (→"S_CARRELLO_PROT35":bool)
            n196 = global read "Globali.vi" "S_TRAZIONE_INSERITA"() -> (→"mA_TRAZIONE_INSERITA":bool)
            n197 = global read "Globali.vi" "C_RESET"() -> (→"C_RESET":bool)
            n198 = global read "Globali.vi" "S_ALLARME_INVERTER"() -> (→"S_ALLARME_INVERTER":bool)
            n199 = global read "Globali.vi" "S_FILTRO_INTASATO_10W30"() -> (→"S_FILTRO_INTASATO_10W30":bool)
            n200 = global read "Globali.vi" "S_FILTRO_INTASATO_W90"() -> (→"S_FILTRO_INTASATO_W90":bool)
            n201 = global read "Globali.vi" "S_PERDITA_10W30"() -> (→"S_PERDITA_10W30":bool)
            n202 = global read "Globali.vi" "S_PERDITA_W90"() -> (→"S_PERDITA_W90":bool)
            n203 = global read "Globali.vi" "S_PRESSOSTATO_ARIA"() -> (→"S_PRESSOSTATO_ARIA":bool)
            n204 = global read "Globali.vi" "S_PERDITA_PROT35"() -> (→"S_PERDITA_PROT35":bool)
            n205 = global read "Globali.vi" "ACCENSIONE_AZIONAMENTO"() -> (→"ACCENSIONE_AZIONAMENTO":bool)
            n206 = global read "Globali.vi" "POMPA_RICIRCOLO"() -> (→"POMPA_RICIRCOLO":bool)
            n207 = global read "Globali.vi" "SBLOCCO_CANCELLI"() -> (→"SBLOCCO_CANCELLI":bool)
            n208 = global read "Globali.vi" "LAMPADA_TRAZIONE_ON"() -> (→"LAMPADA_TRAZIONE_ON":bool)
            n209 = global read "Globali.vi" "LAMPADA_GIALLA"() -> (→"LAMPADA_GIALLA":bool)
            n210 = global read "Globali.vi" "CICALINO"() -> (→"CICALINO":bool)
            n211 = global read "Globali.vi" "RICIRCOLO_OLIO"() -> (→"RICIRCOLO_OLIO":bool)
            n212 = global read "Globali.vi" "CHIUSURA_CANCELLI"() -> (→"CHIUSURA_CANCELLI":bool)
            n213 = global read "Globali.vi" "POMPA_10W30"() -> (→"POMPA_10W30":bool)
            n214 = global read "Globali.vi" "POMPA_W90"() -> (→"POMPA_W90":bool)
            n215 = global read "Globali.vi" "LAMPADA_ROSSA"() -> (→"LAMPADA_ROSSA":bool)
            n216 = global read "Globali.vi" "S_MAN"() -> (→"S_MAN":bool)
            n217 = global read "Globali.vi" "S_TERMICA_RICIRCOLO"() -> (→"S_TERMICA_RICIRCOLO":bool)
            n218 = global read "Globali.vi" "CARICO_ARIA_6_BAR"() -> (→"CARICO_ARIA_6_BAR":bool)
            n219 = global read "Globali.vi" "CALIBRAZIONE_TORSIOMETRO"() -> (→"CALIBRAZIONE_TORSIOMETRO":bool)
            n220 = global read "Globali.vi" "SCARICO_A"() -> (→"SCARICO_A":bool)
            n221 = global read "Globali.vi" "SCARICO_B"() -> (→"SCARICO_B":bool)
            n222 = global read "Globali.vi" "POMPA_PROT35"() -> (→"POMPA_PROT35":bool)
            n223 = global read "Globali.vi" "LAMPADA_VERDE"() -> (→"LAMPADA_VERDE":bool)
            n224 = global read "Globali.vi" "SCARICO_ARIA_6_BAR"() -> (→"SCARICO_ARIA_6_BAR":bool)
            n225 = global read "Globali.vi" "APERTURA_CANCELLI"() -> (→"APERTURA_CANCELLI":bool)
            n226 = global read "Globali.vi" "EROGAZIONE_10W30"() -> (→"EROGAZIONE_10W30":bool)
            n227 = global read "Globali.vi" "EROGAZIONE_W90"() -> (→"EROGAZIONE_W90":bool)
            n228 = global read "Globali.vi" "EROGAZIONE_PROT35"() -> (→"EROGAZIONE_PROT35":bool)
            n229 = global read "Globali.vi" "ROTAZIONE_SX"() -> (→"ROTAZIONE_SX":bool)
            n230 = global read "Globali.vi" "S_AUTO"() -> (→"S_AUTO":bool)
            n231 = global read "Globali.vi" "S_PAUSA"() -> (→"S_PAUSA":bool)
            n232 = global read "Globali.vi" "S_TERMICA_10W30"() -> (→"S_TERMICA_10W30":bool)
            n233 = global read "Globali.vi" "S_TERMICA_W90"() -> (→"S_TERMICA_W90":bool)
            n234 = global read "Globali.vi" "S_TERMICA_PROT35"() -> (→"S_TERMICA_PROT35":bool)
            n235 = global read "Globali.vi" "S_FILTRO_INTASATO_RICIRC"() -> (→"S_FILTRO_INTASATO_RICIRC":bool)
            n236 = global read "Globali.vi" "CARICO_PRESSURIZZ"() -> (→"CARICO_PRESSURIZZ":bool)
            n237 = global read "Globali.vi" "START_MOTORE"() -> (→"START_MOTORE":bool)
            n238 = global read "Globali.vi" "S_FILTRO_INTASATO_PROT35"() -> (→"S_FILTRO_INTASATO_PROT35":bool)
            n239 = global read "Globali.vi" "SCARICO_PRESSURIZZ"() -> (→"SCARICO_PRESSURIZZ":bool)
            n240 = local write "Uscita"("Uscita") -> ()
            n241 = Build Array("Uscita") -> (w331:bool[])
            n242 = call "Cambio Pagina.vi"("pagina in"=w330, "pulsanti"=w331) -> ("pagina out"=→"pagina out":u8, "premuto"=w329:bool)
            n243 = global read "Globali.vi" "stop"() -> (w335:bool)
            n244 = Not(x=w329) -> (.not. x?=w328:bool)
            n245 = Compound Arithmetic op=OR(w335, w328) -> (w334:bool)
            n246 = global read "Globali.vi" "mA_GONFIAGGIO_OK"() -> (→"mA_GONFIAGGIO_OK":bool)
            n247 = global read "Globali.vi" "mA_RICIRCOLO_OK"() -> (→"mA_RICIRCOLO_OK":bool)
            n248 = global read "Globali.vi" "mA_RISCALDAMENTO_OK"() -> (→"mA_RISCALDAMENTO_OK":bool)
            n249 = global read "Globali.vi" "mA_RODAGGIO_OK"() -> (→"mA_RODAGGIO_OK":bool)
            n250 = global read "Globali.vi" "mA_COPPIA_1_FUN_OK"() -> (→"mA_COPPIA_1_FUN_OK":bool)
            n251 = global read "Globali.vi" "mA_COPPIA_2_FUN_OK"() -> (→"mA_COPPIA_2_FUN_OK":bool)
            n252 = global read "Globali.vi" "mA_COPPIA_3_FUN_OK"() -> (→"mA_COPPIA_3_FUN_OK":bool)
            n253 = global read "Globali.vi" "mA_COPPIA_4_FUN_OK"() -> (→"mA_COPPIA_4_FUN_OK":bool)
            n254 = global read "Globali.vi" "mA_COPPIA_5_FUN_OK"() -> (→"mA_COPPIA_5_FUN_OK":bool)
            n255 = global read "Globali.vi" "mA_RICIRCOLO_1_FUN_OK"() -> (→"mA_RICIRCOLO_1_FUN_OK":bool)
            n256 = global read "Globali.vi" "mA_RICIRCOLO_2_FUN_OK"() -> (→"mA_RICIRCOLO_2_FUN_OK":bool)
            n257 = global read "Globali.vi" "mA_RICIRCOLO_3_FUN_OK"() -> (→"mA_RICIRCOLO_3_FUN_OK":bool)
            n258 = global read "Globali.vi" "mA_RICIRCOLO_4_FUN_OK"() -> (→"mA_RICIRCOLO_4_FUN_OK":bool)
            n259 = global read "Globali.vi" "mA_RICIRCOLO_5_FUN_OK"() -> (→"mA_RICIRCOLO_5_FUN_OK":bool)
            n260 = global read "Globali.vi" "PLC->PC"() -> (w276:u16[])
            n261 = global read "Globali.vi" "S_ALLARME"() -> (→"S_ALLARME":bool)
            n262 = global read "Globali.vi" "mA_TRAZIONE_INSERITA"() -> (→"S_TRAZIONE_INSERITA":bool)
            n263 = global read "Globali.vi" "mA_TRAZIONE_DISINSERITA"() -> (→"mA_TRAZIONE_DISINSERITA":bool)
            n264 = global read "Globali.vi" "mA_PERDITE_DX_OK"() -> (→"mA_PERDITE_DX_OK":bool)
            n265 = global read "Globali.vi" "mA_PERDITE_SX_OK"() -> (→"mA_PERDITE_SX_OK":bool)
            n266 = global read "Globali.vi" "mA_PRESSURIZZ_DX_OK"() -> (→"mA_PRESSURIZZ_DX_OK":bool)
            n267 = global read "Globali.vi" "mA_PRESSURIZZ_SX_OK"() -> (→"mA_PRESSURIZZ_SX_OK":bool)
            n268 = global read "Globali.vi" "mA_PRESS_INSERZ_ASSE_OK"() -> (→"mA_PRESS_INSERZ_ASSE_OK":bool)
            n269 = global read "Globali.vi" "mA_PRESS_PRESSURIZZ_OK"() -> (→"mA_PRESS_PRESSURIZZ_OK":bool)
            n270 = Number To Decimal String(number=w276) -> (decimal integer string=w273:string[])  [unwired: 1 in]
            n271 = Array Subset(array=w273, index=0, length=32) -> (w290:string[])
            n272 = Array Subset(array=w273, index=32, length=32) -> (w288:string[])
            n273 = Array Subset(array=w273, index=64, length=32) -> (w286:string[])
            n274 = Array Subset(array=w273, index=96, length=32) -> (w284:string[])
            n275 = Array Subset(array=w273, index=128, length=32) -> (w282:string[])
            n276 = Array Subset(array=w273, index=160, length=32) -> (w278:string[])
            n277 = Array Subset(array=w275, index=0, length=32) -> (w298:string[])
            n278 = Array Subset(array=w275, index=32, length=32) -> (w289:string[])
            n279 = Array Subset(array=w275, index=64, length=32) -> (w287:string[])
            n280 = Array Subset(array=w275, index=96, length=32) -> (w285:string[])
            n281 = Array Subset(array=w275, index=128, length=32) -> (w283:string[])
            n282 = Array Subset(array=w275, index=160, length=32) -> (w277:string[])
            n283 = Replace Array Subset(array=string[][] [["", "", "", "", "", "", "", "", "", "", "", "", "", "", "", "", "", "", "", "", "", "", "", "", "", "", "", "", "", "", "", "", "", "", "", "", "", "", "", "", "", "", "", "", "", "", "", "", "", "", "", "", "", "", "", "", "", "", "", "", "", "", "", "", "", "", "", "", "", "", "", "", "", "", "", "", "", "", "", "", "", "", "", "", "", "", "", "", "", "", "", "", "", "", "", "", "", "", "", "", "", "", "", "", "", "", "", "", "", "", "", "", "", "", "", "", "", "", "", "", "", "", "", "", "", "", "", ""], ["", "", "", "", "", "", "", "", "", "", "", "", "", "", "", "", "", "", "", "", "", "", "", "", "", "", "", "", "", "", "", "", "", "", "", "", "", "", "", "", "", "", "", "", "", "", "", "", "", "", "", "", "", "", "", "", "", "", "", "", "", "", "", "", "", "", "", "", "", "", "", "", "", "", "", "", "", "", "", "", "", "", "", "", "", "", "", "", "", "", "", "", "", "", "", "", "", "", "", "", "", "", "", "", "", "", "", "", "", "", "", "", "", "", "", "", "", "", "", "", "", "", "", "", "", "", "", ""], ["", "", "", "", "", "", "", "", "", "", "", "", "", "", "", "", "", "", "", "", "", "", "", "", "", "", "", "", "", "", "", "", "", "", "", "", "", "", "", "", "", "", "", "", "", "", "", "", "", "", "", "", "", "", "", "", "", "", "", "", "", "", "", "", "", "", "", "", "", "", "", "", "", "", "", "", "", "", "", "", "", "", "", "", "", "", "", "", "", "", "", "", "", "", "", "", "", "", "", "", "", "", "", "", "", "", "", "", "", "", "", "", "", "", "", "", "", "", "", "", "", "", "", "", "", "", "", ""], ["", "", "", "", "", "", "", "", "", "", "", "", "", "", "", "", "", "", "", "", "", "", "", "", "", "", "", "", "", "", "", "", "", "", "", "", "", "", "", "", "", "", "", "", "", "", "", "", "", "", "", "", "", "", "", "", "", "", "", "", "", "", "", "", "", "", "", "", "", "", "", "", "", "", "", "", "", "", "", "", "", "", "", "", "", "", "", "", "", "", "", "", "", "", "", "", "", "", "", "", "", "", "", "", "", "", "", "", "", "", "", "", "", "", "", "", "", "", "", "", "", "", "", "", "", "", "", ""], ["", "", "", "", "", "", "", "", "", "", "", "", "", "", "", "", "", "", "", "", "", "", "", "", "", "", "", "", "", "", "", "", "", "", "", "", "", "", "", "", "", "", "", "", "", "", "", "", "", "", "", "", "", "", "", "", "", "", "", "", "", "", "", "", "", "", "", "", "", "", "", "", "", "", "", "", "", "", "", "", "", "", "", "", "", "", "", "", "", "", "", "", "", "", "", "", "", "", "", "", "", "", "", "", "", "", "", "", "", "", "", "", "", "", "", "", "", "", "", "", "", "", "", "", "", "", "", ""], ["", "", "", "", "", "", "", "", "", "", "", "", "", "", "", "", "", "", "", "", "", "", "", "", "", "", "", "", "", "", "", "", "", "", "", "", "", "", "", "", "", "", "", "", "", "", "", "", "", "", "", "", "", "", "", "", "", "", "", "", "", "", "", "", "", "", "", "", "", "", "", "", "", "", "", "", "", "", "", "", "", "", "", "", "", "", "", "", "", "", "", "", "", "", "", "", "", "", "", "", "", "", "", "", "", "", "", "", "", "", "", "", "", "", "", "", "", "", "", "", "", "", "", "", "", "", "", ""], ["", "", "", "", "", "", "", "", "", "", "", "", "", "", "", "", "", "", "", "", "", "", "", "", "", "", "", "", "", "", "", "", "", "", "", "", "", "", "", "", "", "", "", "", "", "", "", "", "", "", "", "", "", "", "", "", "", "", "", "", "", "", "", "", "", "", "", "", "", "", "", "", "", "", "", "", "", "", "", "", "", "", "", "", "", "", "", "", "", "", "", "", "", "", "", "", "", "", "", "", "", "", "", "", "", "", "", "", "", "", "", "", "", "", "", "", "", "", "", "", "", "", "", "", "", "", "", ""], ["", "", "", "", "", "", "", "", "", "", "", "", "", "", "", "", "", "", "", "", "", "", "", "", "", "", "", "", "", "", "", "", "", "", "", "", "", "", "", "", "", "", "", "", "", "", "", "", "", "", "", "", "", "", "", "", "", "", "", "", "", "", "", "", "", "", "", "", "", "", "", "", "", "", "", "", "", "", "", "", "", "", "", "", "", "", "", "", "", "", "", "", "", "", "", "", "", "", "", "", "", "", "", "", "", "", "", "", "", "", "", "", "", "", "", "", "", "", "", "", "", "", "", "", "", "", "", ""]] ("PLC->PC"), new element #1=w298, index (row) #1=0 ("index (row)"), new element #2=w290, index (row) #2=1 ("index (row)"), new element #3=w289, index (row) #3=2 ("index (row)"), new element #4=w288, index (row) #4=3 ("index (row)"), new element #5=w287, index (row) #5=4 ("index (row)"), new element #6=w286, index (row) #6=5 ("index (row)"), new element #7=w285, index (row) #7=6 ("index (row)"), new element #8=w284, index (row) #8=7 ("index (row)"), new element #9=w283, index (row) #9=8 ("index (row)"), new element #10=w282, index (row) #10=9 ("index (row)"), new element #11=w277, index (row) #11=10 ("index (row)"), new element #12=w278, index (row) #12=11 ("index (row)")) -> (w299:string[][])  [unwired: 12 in]
            n284 = Transpose 2D Array(2D array=w299) -> (transposed array=→"PLC->PC":string[][])
          }
          n285 = node-c288(w24) -> ()  [unwired: 1 out]
        }
        frame Error {
        }
      }
      "error out (no error)" <- w22
    }
    frame #1 {
      n286 = local write "Uscita"(FALSE ("Pag. collaudo")) -> ()
    }
  }
  n287 = To Upper Case(1:"Pagina diagnostica" ("Errore conn. centralina")) -> (0:→"Errore conn. centralina":string)
